vi "Data_Condition.vi"(2 "Voltage IN":T1, 3 "Current IN":T1) -> (0 "Voltage_Out":dbl[][](array[numeric]), 1 "Current_Out":dbl[][](array[numeric]))   [LabVIEW 2018]
uses:
  <vilib>/Analysis/Matrix/Datatypes/RealMatrix.ctl
  <vilib>/Analysis/Matrix/NI_Matrix.lvlib
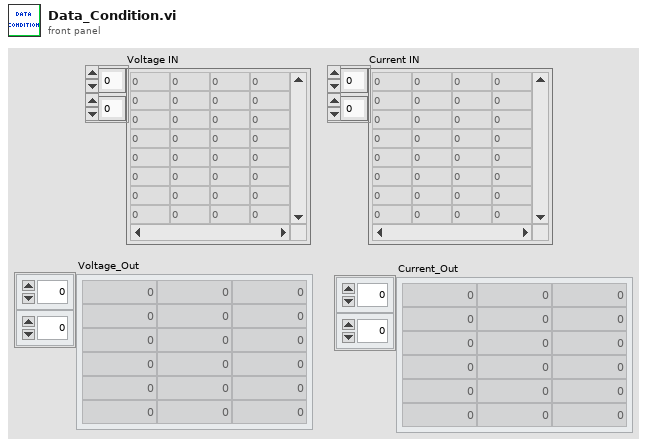
[diagram p1: front panel]
types:
  T1 = typedef "NI_Matrix.lvlib/RealMatrix.ctl" = dbl[][]
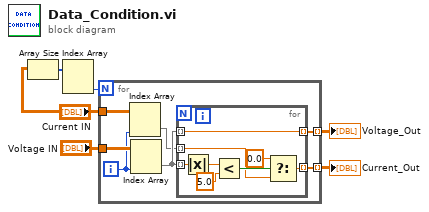
[diagram p0: block diagram]
diagram:
  n1 = Array Size(array="Current IN") -> (size(s)=w6:i32[])
  n2 = Index Array(array=w6) -> (element #2=w5:i32)  [unwired: 2 in, 1 out]
  n3 = for {
    N: w5 -> [_]
    tunnel: "Current IN" -> [w13]
    tunnel: "Voltage IN" -> [w12]
    tunnel: [w8] -> w2 mode=indexing
    tunnel: [w7] -> w1 mode=indexing
    i -> [w11]
    n4 = Index Array(array=w13, index (col)=w11) -> (element=w9:dbl[])  [unwired: 1 in]
    n5 = Index Array(array=w12, index (col)=w11) -> (element=w10:dbl[])  [unwired: 1 in]
    n6 = for {
      tunnel: w10 -> [w19] mode=indexing
      tunnel: w10 -> [w16] mode=indexing
      tunnel: w9 -> [w15] mode=indexing
      tunnel: [w17] -> w7 mode=indexing
      tunnel: [w16] -> w8 mode=indexing
      n7 = Absolute Value(x=w19) -> (abs(x)=w21:dbl)
      n8 = Less?(x=w21, y=5.0) -> (x < y?=w18:bool)
      n9 = Select(t=0.0, s=w18, f=w15) -> (s? t:f=w17:dbl)
    }
  }
  "Voltage_Out" <- w2
  "Current_Out" <- w1
